vi "Test IBW.vi"() -> ()   [LabVIEW 2019]
panel:
  out "Average Time":dbl
  # "Old = 0.152405\nNew = 0.0112605"
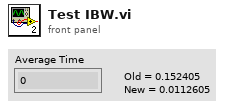
[diagram p1: front panel]
types:
  T1 = typedef "IMAQ Image.ctl" = refnum<image>
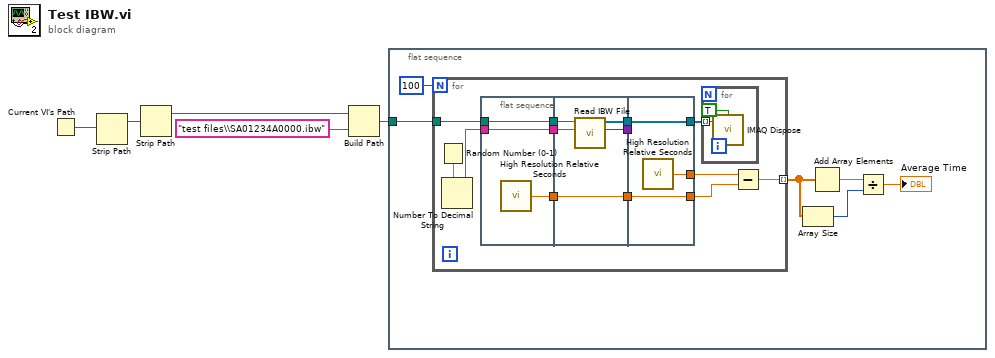
[diagram p0: block diagram]
diagram:
  n1 = Current VI's Path() -> (path=w5:path)
  n2 = Strip Path(path=w5) -> (stripped path=w4:path)  [unwired: 1 out]
  n3 = Strip Path(path=w4) -> (stripped path=w3:path)  [unwired: 1 out]
  n4 = Build Path(base path=w3, name or relative path="test files\\SA01234A0000.ibw") -> (appended path=w1:path)
  n5 = flat-sequence {
    tunnel: w1 -> [w6]
    frame #0 {
      n6 = for {
        N: 100 -> [_]
        tunnel: [w20] -> w10 mode=indexing
        tunnel: w6 -> [w18]
        n7 = Random Number (0-1)() -> (number: 0 to 1=w16:dbl)
        n8 = Number To Decimal String(number=w16) -> (decimal integer string=w14:string)  [unwired: 1 in]
        n9 = flat-sequence {
          tunnel: [w29] -> w23
          tunnel: [w28] -> w19
          tunnel: w18 -> [w28]
          tunnel: [w27] -> w15
          tunnel: w14 -> [w27]
          tunnel: w23 -> [w34]
          tunnel: [w34] -> w22
          tunnel: w19 -> [w33]
          tunnel: [w32] -> w17
          tunnel: w15 -> [w31]
          tunnel: [w30] -> w12
          tunnel: [w37] -> w24
          tunnel: w22 -> [w36]
          tunnel: [w36] -> w21
          tunnel: w17 -> [_]
          tunnel: [w35] -> w13
          tunnel: w12 -> [w35]
          frame #0 {
            n10 = call <vilib>:"High Resolution Relative Seconds.vi"() -> ("relative seconds"=w29:dbl)
          }
          frame #1 {
            n11 = call "Read IBW File.vi"("Basename"=w31, "Path"=w33) -> ("Notes LUT"=w32:variant, "IMAQ"=w30:T1[])  [unwired: 7 in, 1 out]
          }
          frame #2 {
            n12 = call <vilib>:"High Resolution Relative Seconds.vi"() -> ("relative seconds"=w37:dbl)
          }
        }
        n13 = for {
          tunnel: w13 -> [w26] mode=indexing
          n14 = call "IMAQ Dispose"("All Images? (No)"=TRUE, "Image"=w26) -> ()  [unwired: 4 in, 1 out]
        }
        n15 = Subtract(x=w24, y=w21) -> (x-y=w20:dbl)
      }
      n16 = Array Size(array=w10) -> (size(s)=w8:i32)
      n17 = Add Array Elements(numeric array=w10) -> (sum=w9:dbl)
      n18 = Divide(x=w9, y=w8) -> (x/y=→"Average Time":dbl)
    }
  }
